vi "Configure Signal Standard.vi"(0 "VISA resource name":refnum<visa-resource-name>, 1 "Signal Operation Type (0: Select Standard)":u16(ring) items=["Select  Standard", "Load Standard"], 5 "Standard Name (0:Off)":i32(ring) items=["Off", "3GPP W-CDMA Downlink", "3GPP W-CDMA Uplink", "Mobile WiMAX (IEEE802.16e) Downlink", "Mobile WiMAX (IEEE802.16e) Uplink", "3GPP LTE Downlink", "3GPP LTE Uplink", "ARIB STD-T75", "3GPP TDD 1.28Mcps Option", "XG-PHS", "3GPP2 CDMA2000 Forward Link", "3GPP2 EV-DO Forward Link", "3GPP LTE TDD Downlink", "3GPP LTE TDD Uplink", "ISDB-Tmm", "WLAN (IEEE802.11)", "ISDB-T", "LR-WPANs (IEEE802.15.4)", "APCO P25", "Microlink ETSI", "NXDN"], 7 "Measurement (0:Adjacent Channel Power)":i32(ring) items=["Adjacent Channel Power", "Channel Power", "Occupied BW", "Burst Average", "Spectrum Emission Mask"], 9 "Signal Standard Setting (0:None)":i32(ring) items=["None", "WCDMA Uplink", "WCDMA Downlink", "WCDMA UL Mean", "WCDMA DL Mean", "WCDMA RRC Filtered", "WCDMA Single Carrier", "WCDMA Two Carrier", "WCDMA Three Carrier", "WCDMA Four Carrier", "WCDMA SEM Uplink Additional", "WCDMA SEM DL  P >= 43dBm", "WCDMA SEM DL  39 dBm <= P < 43dBm", "WCDMA SEM DL  31 dBm <= P < 39dBm", "WCDMA SEM DL  P < 31 dBm", "WCDMA SEM DL  P >= 43dBm Additional", "WCDMA SEM DL  39 dBm <= P < 43dBm Additional", "WCDMA SEM DL  31 dBm <= P < 39dBm Additional", "Mobile WiMAX 5MHz BW", "Mobile WiMAX 10MHz BW", "Mobile WiMAX 5ms Frame", "LTE 1.4MHz BW", "LTE 3MHz BW", "LTE 5MHz BW", "LTE 10MHz BW", "LTE 15MHz BW", "LTE 20MHz BW", "LTE 1.4MHz BW 5MHz UTRA", "LTE 1.4MHz BW 1.4MHz E-UTRA ", "LTE 3MHz BW 5MHz UTRA", "LTE 3MHz BW 3MHz E-UTRA", "LTE 5MHz BW 5MHz UTRA", "LTE 5MHz BW 5MHz E-UTRA", "LTE 10MHz BW 5MHz UTRA", "LTE 10MHz BW 10MHz E-UTRA", "LTE 15MHz BW 5MHz UTRA", "LTE 15MHz BW 15MHz E-UTRA", "LTE 20MHz BW 5MHz UTRA", "LTE 20MHz BW 20MHz E-UTRA", "LTE Mean Power 1.4MHz BW ", "LTE Mean Power 3MHz BW", "LTE Mean Power 5MHz BW", "LTE Mean Power 10MHz BW", "LTE Mean Power 15MHz BW", "LTE Mean Power 20MHz BW", "LTE Filtered Power 1.4MHz BW", "LTE Filtered Power 3MHz BW", "LTE Filtered Power 5MHz BW", "LTE Filtered Power 10MHz BW", "LTE Filtered Power 15MHz BW", "LTE Filtered Power 20MHz BW", "ETC-DSRC Pi/4 DQPSK", "ETC-DSRC ASK", "ETC-DSRC Mean Power", "TD-SCDMA Single Carrier", "TD-SCDMA Two Carriers", "TD-SCDMA Three Carriers", "TD-SCDMA Four Carriers", "TD-SCDMA Five Carriers", "TD-SCDMA Six Carriers", "TD-SCDMA TDD 1.28Mcps", "TD-SCDMA 5ms Subframe", "TD-SCDMA DL Trace Point Tune 34dBm<=P", "TD-SCDMA DL Trace Point Tune 26dBm<=P<34dBm", "TD-SCDMA DL Trace Point Tune P<26dBm", "TD-SCDMA UL Trace Point Tune -53.5dBm<=P", "TD-SCDMA UL Trace Point Tune -55dBm<=P", "TD-SCDMA DL Actual 34 dBm <= P", "TD-SCDMA DL Actual 26 dBm <= P < 34 dBm", "TD-SCDMA DL Actual P < 26 dBm", "TD-SCDMA UL Actual -53.5 dBm <= P", "TD-SCDMA UL Actual -55 dBm <= P", "TD-SCDMA DL Fast 34 dBm <= P", "TD-SCDMA DL Fast 26 dBm <= P < 34 dBm", "TD-SCDMA DL Fast P < 26 dBm ", "TD-SCDMA UL Fast -53.5 dBm <= P", "TD-SCDMA UL Fast -55 dBm <= P", "XG-PHS (OBW Measurement) 10MHz BW", "XG-PHS (OBW Measurement) 20MHz BW", "XG-PHS (CHP Measurement) Mean Power 10MHz BW", "XG-PHS (CHP Measurement) Mean Power 20MHz BW", "XG-PHS (SEM) Base station channel interval: 10MHz BW", "XG-PHS (SEM) Mobile station channel interval: 10MHz BW"], 11 "error in (no error)":errorcluster) -> (4 "VISA resource name out":refnum<visa-resource-name>, 15 "error out":errorcluster)   [LabVIEW 2020, in "Anritsu Signal Analyzer Series.lvlib"]
doc: "Configures the signal standard operation, name and setting according to Measurement selected."
uses:
  Anritsu Signal Analyzer Series.lvlib
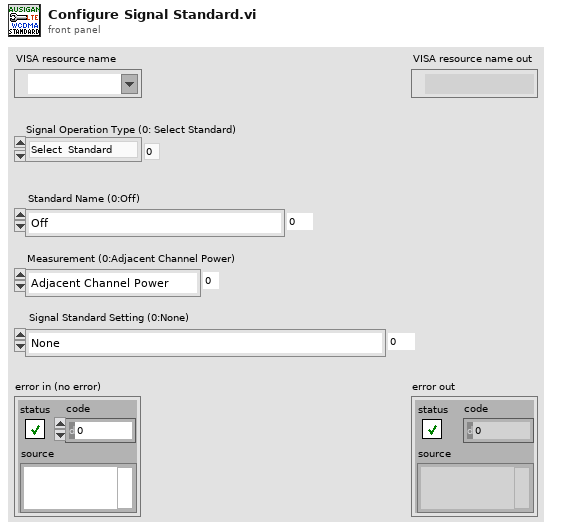
[diagram p1: front panel]
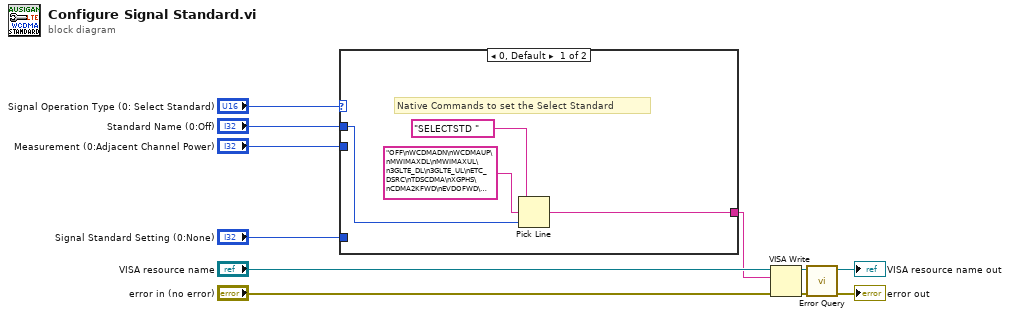
[diagram p0: block diagram]
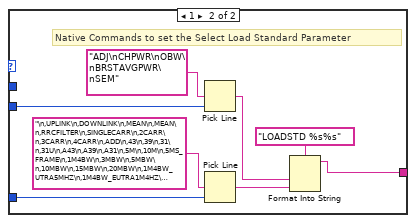
[diagram p2: hidden frame]
diagram:
  n1 = case shown="0, Default" "Signal Operation Type (0: Select Standard)" {
    tunnel: "Measurement (0:Adjacent Channel Power)" -> [_ w23]
    tunnel: [w12 w21] -> w4
    tunnel: "Signal Standard Setting (0:None)" -> [_ w18]
    tunnel: "Standard Name (0:Off)" -> [w13 _]
    frame 0, Default {
      # "Native Commands to set the Select Standard"
      n2 = Pick Line(string ("")="SELECTSTD " ("_CommandSet"), multi-line string="OFF\nWCDMADN\nWCDMAUP\nMWIMAXDL\nMWIMAXUL\n3GLTE_DL\n3GLTE_UL\nETC_DSRC\nTDSCDMA\nXGPHS\nCDMA2KFWD\nEVDOFWD\n3GLTE_TDD_DL\n3GLTE_TDD_UL\nISDBTMM\nWLAN\nISDBT\nLRWPANS\nAPCO_P25\nMICROLINKETSI\nNXDN" ("String"), line index=w13) -> (output string=w12:string)
    }
    frame 1 {
      # "Native Commands to set the Select Load Standard Parameter"
      n3 = Pick Line(multi-line string="ADJ\nCHPWR\nOBW\nBRSTAVGPWR\nSEM" ("複数行文字列"), line index=w23) -> (output string=w19:string)  [unwired: 1 in]
      n4 = Pick Line(multi-line string="\n,UPLINK\n,DOWNLINK\n,MEAN\n,MEAN\n,RRCFILTER\n,SINGLECARR\n,2CARR\n,3CARR\n,4CARR\n,ADD\n,43\n,39\n,31\n,31U\n,A43\n,A39\n,A31\n,5M\n,10M\n,5MS_FRAME\n,1M4BW\n,3MBW\n,5MBW\n,10MBW\n,15MBW\n,20MBW\n,1M4BW_UTRA5MHZ\n,1M4BW_EUTRA1M4HZ\n,3MBW_UTRA5MHZ\n,3MBW_EUTRA3MHZ\n,5MBW_UTRA5MHZ\n,5MBW_EUTRA5MHZ\n,10MBW_UTRA5MHZ\n,10MBW_EUTRA10MHZ\n,15MBW_UTRA5MHZ\n,15MBW_EUTRA15MHZ\n,20MBW_UTRA5MHZ\n,20MBW_EUTRA20MHZ\n,MEAN_1M4BW\n,MEAN_3MBW\n,MEAN_5MBW\n,MEAN_10MBW\n,MEAN_15MBW\n,MEAN_20MBW\n,FILTERED_1M4BW\n,FILTERED_3MBW\n,FILTERED_5MBW\n,FILTERED_10MBW\n,FILTERED_15MBW\n,FILTERED_20MBW\n,PI4DQPSK\n,ASK\n,MEAN\n,TDD128M1C\n,TDD128M2C\n,TDD128M3C\n,TDD128M4C\n,TDD128M5C\n,TDD128M6C\n,TDD128M\n,MEAN\n,DLT34\n,DLT26\n,DLT26U\n,ULT53\n,ULT55\n,DL34\n,DL26\n,DL26U\n,UL53\n,UL55\n,DLF34\n,DLF26\n,DLF26U\n,ULF53\n,ULF55\n,10MBW\n,20MBW\n,MEAN_10MBW\n,MEAN_20MBW\n,BS_10MBW\n,UE_10MBW" ("文字列"), line index=w18) -> (output string=w16:string)  [unwired: 1 in]
      n5 = Format Into String(format string="LOADSTD %s%s" ("_Command"), w19, w16) -> (resulting string=w21:string)  [unwired: 2 in, 1 out]
    }
  }
  n6 = VISA Write(VISA resource name="VISA resource name", write buffer=w4, error in (no error)="error in (no error)") -> (VISA resource name out=w5:refnum<visa-resource-name>, error out=w6:errorcluster)  [unwired: 1 out]
  n7 = call "Error Query.vi"("error in (no error)"=w6, "VISA resource name"=w5) -> ("error out"=→"error out":errorcluster, "VISA resource name out"=→"VISA resource name out":refnum<visa-resource-name>)  [unwired: 6 in, 2 out]
